vi "Instrument Status.vi"(8 "error in (no error)":errorcluster, 11 "VISA resource name":refnum<visa-resource-name>) -> (0 "error out":errorcluster, 2 "Lock Code":u16=123, 3 "VISA resource name out":refnum<visa-resource-name>, 4 "Remote Interface Mode":u16(ring) items=["Local", "Remote", "Remote with local lockout"], 5 "Keypad Locked?":bool)   [LabVIEW 2024, in "Lake Shore 336.lvlib"]
doc: "This VI returns various instrument settings. Parameters returned are;\nRemote interface mode, key status, and keypad lock out."
uses:
  Lake Shore 336.lvlib
  Instance           1 25Saved   Instrument Status .vi
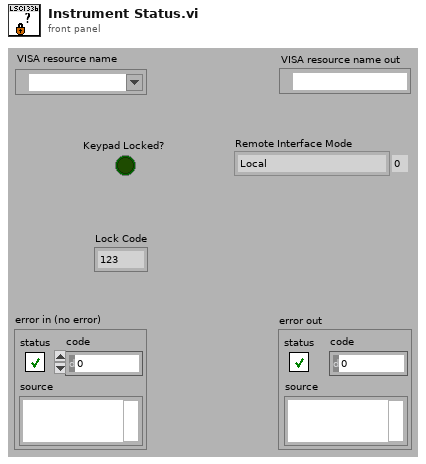
[diagram p1: front panel]
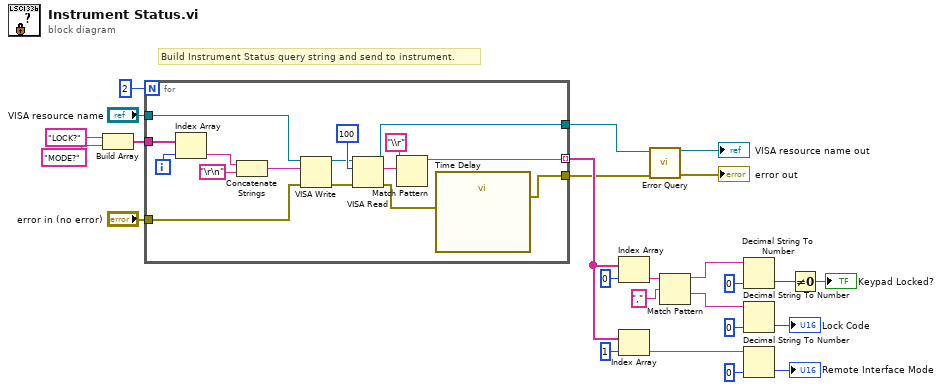
[diagram p0: block diagram]
diagram:
  # "Build Instrument Status query string and send to instrument."
  n1 = Build Array("LOCK?", "MODE?") -> (w23:string[])
  n2 = for {
    N: 2 -> [_]
    tunnel: [w35] -> w1
    tunnel: [w30] -> w2
    tunnel: "VISA resource name" -> [w34]
    tunnel: "error in (no error)" -> [w33]
    tunnel: w23 -> [w32]
    tunnel: [w31] -> w16 mode=indexing
    i -> [w36]
    n3 = Index Array(array=w32, index=w36) -> (element=w26:string)
    n4 = Concatenate Strings(w26, "\r\n") -> (w27:string)
    n5 = VISA Write(VISA resource name=w34, write buffer=w27, error in (no error)=w33) -> (VISA resource name out=w38:refnum<visa-resource-name>, error out=w37:errorcluster)  [unwired: 1 out]
    n6 = VISA Read(VISA resource name=w38, byte count=100, error in (no error)=w37) -> (VISA resource name out=w35:refnum<visa-resource-name>, read buffer=w40:string, error out=w29:errorcluster)  [unwired: 1 out]
    n7 = Match Pattern(string=w40, regular expression="\\r") -> (before substring=w31:string)  [unwired: 1 in, 3 out]
    n8 = call "Time Delay"("error in (no error)"=w29) -> ("error out"=w30:errorcluster)  [unwired: 10 in]
  }
  n9 = Index Array(array=w16, index=0) -> (element=w18:string)
  n10 = Index Array(array=w16, index=1) -> (element=w14:string)
  n11 = call "Error Query.vi"("error in (no error)"=w2, "VISA resource name"=w1) -> ("error out"=→"error out":errorcluster, "VISA resource name out"=→"VISA resource name out":refnum<visa-resource-name>)  [unwired: 7 in, 1 out]
  n12 = Match Pattern(string=w18, regular expression=",") -> (before substring=w9:string, after substring=w8:string)  [unwired: 1 in, 2 out]
  n13 = Decimal String To Number(string=w9, default (0L)=u16 0) -> (number=w10:u16)  [unwired: 1 in, 1 out]
  n14 = Decimal String To Number(string=w8, default (0L)=u16 0) -> (number=→"Lock Code":u16)  [unwired: 1 in, 1 out]
  n15 = Decimal String To Number(string=w14, default (0L)=u16 0) -> (number=→"Remote Interface Mode":u16)  [unwired: 1 in, 1 out]
  n16 = Not Equal To 0?(x=w10) -> (x != 0?=→"Keypad Locked?":bool)
